vi "Front Panel.vi"(11 "GUI In":refnum<class "PAS Derived.lvclass">) -> ()   [LabVIEW 2015, in "PAS Derived.lvclass"]
uses:
  PAS Derived.lvclass
  Reusable/Xctls/Buffer/2D Control/2D Buffer Display.xctl
  Reusable/GUI/GUI.lvclass/GUI.ctl
  Reusable/Observer/Observer.lvclass/Observer.ctl
  Data/cPAS Data.lvclass
  Reusable/GUI/Accessors/Read RegEvent.vi
  Reusable/Observer/Read Data Queue.vi
  Reusable/PAS/Data/Main/Read CellData.vi
  Reusable/Data/Read measTime.vi
  Reusable/Data/Data.lvclass
  Reusable/PAS/Data/Cell/PAS Cell Data.lvclass
panel:
  out "pasDerData":cluster{"data_out":sgl[][], "time":timestamp}(xcontrol)
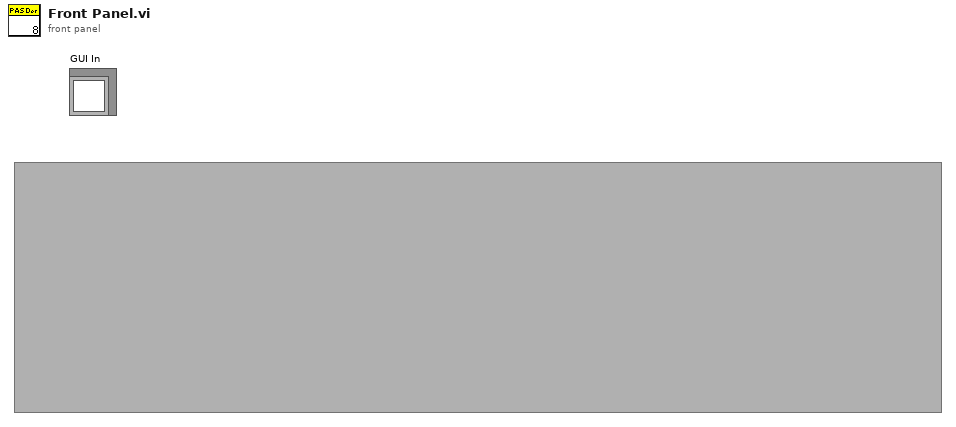
[diagram p1: front panel]
types:
  T1 = cluster{"Name":string, "Line Width":u8, "Line Style":u8, "Color":u32}[]
  T2 = cluster{"f0":sgl, "IA":sgl, "Q":sgl, "max":dbl[], "deltaPhi":dbl, "tau":dbl, "noiseLim":dbl, "ext":dbl}
  T3 = cluster{"f0":sgl, "IA":sgl, "Q":sgl, "max":sgl[], "deltaPhi":sgl, "tau":sgl, "noiseLim":sgl, "ext":sgl}
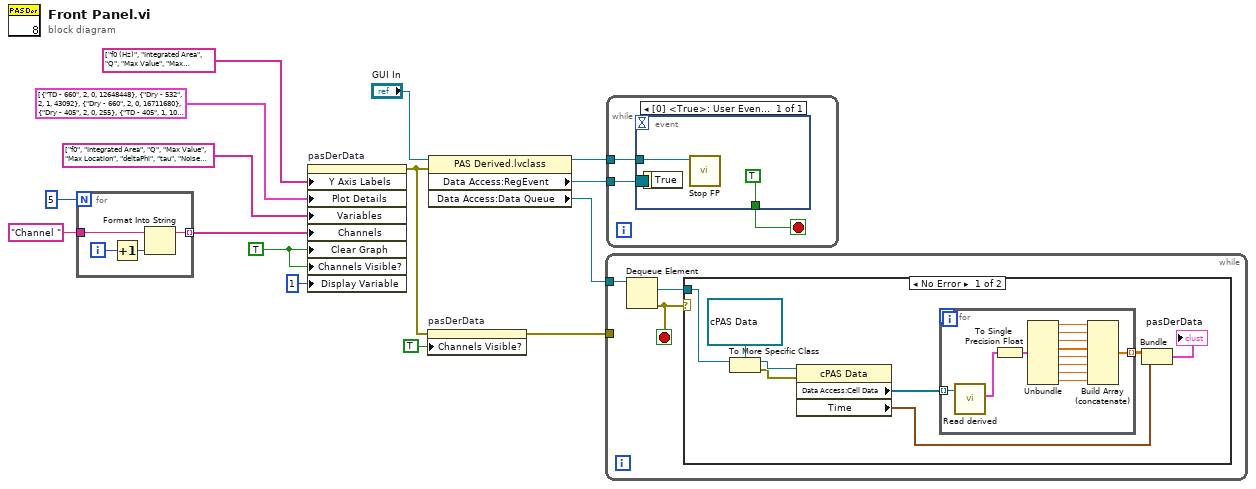
[diagram p0: block diagram]
diagram:
  w5 = TRUE ("Clear Graph")
  n1 = for {
    N: 5 -> [_]
    tunnel: "Channel " -> [w17]
    tunnel: [w16] -> w9 mode=indexing
    i -> [w19]
    n2 = Increment(x=w19) -> (x+1=w18:i32)
    n3 = Format Into String(initial string=w17, w18) -> (resulting string=w16:string)  [unwired: 2 in, 1 out]
  }
  n4 = property on="pasDerData" class="2D Buffer Display (strict)"("Y Axis Labels"=string[] ["f0 (Hz)", "Integrated Area", "Q", "Max Value", "Max Location (Hz)", "delta Phi", "tau", "Noise Limit", "Absorbtion (Mm^-1)"], "Plot Details"=T1 [{"Name"="TD - 660", "Line Width"=2, "Line Style"=0, "Color"=12648448}, {"Name"="Dry - 532", "Line Width"=2, "Line Style"=1, "Color"=43092}, {"Name"="Dry - 660", "Line Width"=2, "Line Style"=0, "Color"=16711680}, {"Name"="Dry - 405", "Line Width"=2, "Line Style"=0, "Color"=255}, {"Name"="TD - 405", "Line Width"=1, "Line Style"=10, "Color"=128}], "Variables"=string[] ["f0", "Integrated Area", "Q", "Max Value", "Max Location", "deltaPhi", "tau", "Noise Limit", "Absorbtion"], "Channels"=w9, "Clear Graph"=w5, "Channels Visible?"=w5, "Display Variable"=1) -> (error out=w2:errorcluster)  [unwired: 2 in, 1 out]
  n5 = property on="pasDerData" class="2D Buffer Display (strict)"(error in=w2, "Channels Visible?"=TRUE) -> (error out=w1:errorcluster)  [unwired: 1 in, 1 out]
  n6 = property class="PAS Derived.lvclass"(reference="GUI In", error in=w2) -> (reference out=w8:refnum<class "PAS Derived.lvclass">, "Data Access:RegEvent"=w15:refnum<event-registration>, "Data Access:Data Queue"=w14:refnum<queue>)  [unwired: 1 out]
  n7 = while {
    tunnel: w14 -> [w22]
    tunnel: w1 -> [_]
    stop <- w21 stop-if-true
    n8 = Dequeue Element(queue=w22) -> (element=w20:refnum<data-value>, error out=w21:errorcluster)  [unwired: 2 in, 2 out]
    n9 = case shown="No Error" w21 {
      tunnel: w20 -> [w30 _]
      frame No Error {
        n10 = To More Specific Class(target class=refnum<data-value> refnum ("data value reference"), reference=w30) -> (specific class reference=w28:refnum<data-value>, error out=w27:errorcluster)  [unwired: 1 in]
        n11 = property class="cPAS Data"(reference=w28, error in=w27) -> ("Data Access:Cell Data"=w26:refnum<class "PAS Cell Data.lvclass">[], "Time"=w24:timestamp)  [unwired: 2 out]
        n12 = for {
          tunnel: w26 -> [w33] mode=indexing
          tunnel: [w31] -> w25 mode=indexing
          n13 = call "Read derived.vi"("PAS Cell Data in"=w33) -> ("derived"=w32:T2)  [unwired: 8 in, 2 out]
          n14 = To Single Precision Float(number=w32) -> (single precision float=w42:T3)
          n15 = Unbundle(w42) -> ("f0"=w40:sgl, "IA"=w34:sgl, "Q"=w41:sgl, "max"=w39:sgl[], "deltaPhi"=w35:sgl, "tau"=w36:sgl, "noiseLim"=w37:sgl, "ext"=w38:sgl)
          n16 = Build Array (concatenate)(w40, w34, w41, w39, w35, w36, w37, w38) -> (w31:sgl[])
        }
        n17 = Bundle(w25, "Time"=w24) -> (→"pasDerData":cluster{sgl[][], "Time":timestamp})  [unwired: 1 in]
      }
      frame Error {
      }
    }
  }
  n18 = while {
    tunnel: w15 -> [w44]
    tunnel: w8 -> [w43]
    stop <- w45 stop-if-true
    n19 = event shown="[0] <True>: User Event" {
      selector: w44 -> [_]
      dyn-events: _ -> [_]
      timeout: _ -> [_]
      tunnel: [TRUE] -> w45
      tunnel: w43 -> [w46]
      event User Event {
        n20 = event-data() -> ()  [unwired: 1 in, 1 out]
        n21 = call-dynamic "Stop FP.vi"("GUI in"=w46) -> ()  [unwired: 9 in, 2 out]
      }
    }
  }
